vi "MoAgSy_Host_GPG_cryption_p.vi"(0 "MoAgSy_Host":refnum<class "MoAgSy_Host.lvclass">, 2 "string in":string, 5 "error IO":errorcluster, 7 "reveicer array":string[](array[string]), 8 "task":enum16{"encrypt", "decrypt", "sign", "verify"}(ring), 9 "receiver":string) -> (13 "success":bool, 14 "dup MoAgSy_Host":refnum<class "MoAgSy_Host.lvclass">, 16 "String out":string, 19 "error out":errorcluster)   [LabVIEW 2009, in "MoAgSy.lvlib" / "MoAgSy_Host.lvclass"]
doc: "use cryption functions with Hosts GPG object\nFunctions:\nEncrypt\nDecrypt\nSign\nVerify\n\nF.Berck@gsi.de\nGSI Darmstadt 2009"
uses:
  MoAgSy_Host.lvclass
  MoAgSy_Host.lvclass/MoAgSy_Host.ctl
  MoAgSy_GPG/MoAgSy_GPG.lvclass
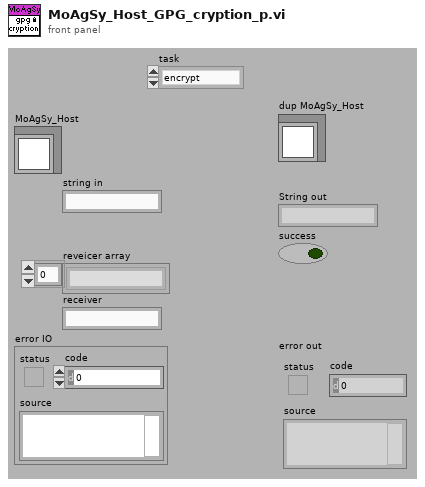
[diagram p1: front panel]
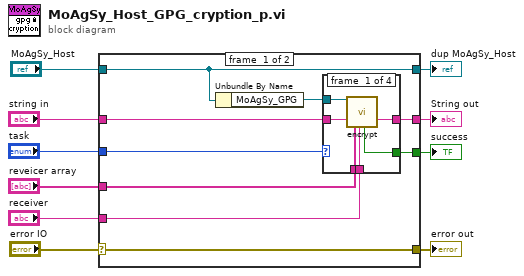
[diagram p0: block diagram]
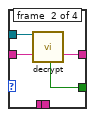
[diagram p2: hidden frame]
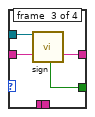
[diagram p3: hidden frame]
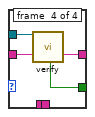
[diagram p4: hidden frame]
diagram:
  n1 = case shown="No Error" "error IO" {
    selector: "error IO" -> [w19 w39]
    tunnel: [w19 w39] -> w10
    tunnel: [w18 w38] -> w9
    tunnel: "MoAgSy_Host" -> [w18 w38]
    tunnel: "string in" -> [w16 _]
    tunnel: "task" -> [w13 _]
    tunnel: "reveicer array" -> [w12 _]
    tunnel: "receiver" -> [w11 _]
    tunnel: [w15 _] -> w4
    tunnel: [w14 _] -> w3
    frame #0 {
      n2 = Unbundle By Name(w18) -> ("MoAgSy_GPG"=w17:refnum<class "MoAgSy_GPG.lvclass">)
      n3 = case shown="\"encrypt\"" w13 {
        tunnel: w17 -> [w25 w29 w33 w36]
        tunnel: w16 -> [w24 w28 w32 w37]
        tunnel: w12 -> [w23 _ _ _]
        tunnel: w11 -> [w22 _ _ _]
        tunnel: [w21 w27 w31 w35] -> w15
        tunnel: [w20 w26 w30 w34] -> w14
        frame #0 {
          n4 = call-dynamic "encrypt.vi"("HGF_GPG"=w25, "string in"=w24, "reveicer array"=w23, "receiver"=w22) -> ("success"=w20:bool, "String out"=w21:string)  [unwired: 5 in, 9 out]
        }
        frame #1 {
          n5 = call-dynamic "decrypt.vi"("HGF_GPG"=w29, "string in"=w28) -> ("success"=w26:bool, "String"=w27:string)  [unwired: 6 in, 10 out]
        }
        frame #2 {
          n6 = call-dynamic "sign.vi"("HGF_GPG"=w33, "string in"=w32) -> ("success"=w30:bool, "String out"=w31:string)  [unwired: 7 in, 9 out]
        }
        frame #3 {
          n7 = call-dynamic "verify.vi"("HGF_GPG"=w36, "string in"=w37) -> ("success"=w34:bool, "String"=w35:string)  [unwired: 5 in, 11 out]
        }
      }
    }
    frame #1 {
    }
  }
  "error out" <- w10
  "dup MoAgSy_Host" <- w9
  "String out" <- w4
  "success" <- w3
